vi "Global.vi"() -> ()   [LabVIEW 2018]
uses:
  Global 1.vi
panel:
  in  "stop":bool
  in  "Boolean":bool
  in  "String":string
  in  "Numeric":dbl
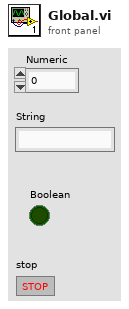
[diagram p1: front panel]
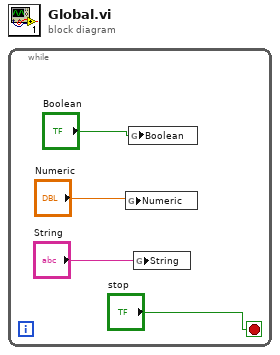
[diagram p0: block diagram]
diagram:
  n1 = while {
    stop <- "stop" stop-if-true
    n2 = global write "Global 1.vi" "Numeric"("Numeric") -> ()
    n3 = global write "Global 1.vi" "Boolean"("Boolean") -> ()
    n4 = global write "Global 1.vi" "String"("String") -> ()
  }
